vi "Pos ctrl window-Build menu.vi"(8 "error in (no error)":errorcluster) -> (0 "error out":errorcluster, 3 "menu reference out":refnum<k9>)   [LabVIEW 2013]
uses:
  Globals/Pos ctrl window globals.vi
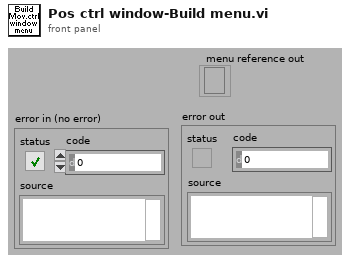
[diagram p1: front panel]
types:
  T1 = typedef "Pos Ctrl window refs cluster.ctl" = cluster{"menu reference":refnum<k9>, "X Coordinate ctrl":refnum<vi>, "Y Coordinate ctrl":refnum<vi>, "Z Coordinate ctrl":refnum<vi>, "Speed setting ctrl":refnum<vi>, "Up":refnum<vi>, "Down":refnum<vi>, "Left":refnum<vi>, "Right":refnum<vi>, "Z move up":refnum<vi>, "Z move down":refnum<vi>, "Down-left":refnum<vi>, "Down-right":refnum<vi>, "Up-left":refnum<vi>, "Up-right":refnum<vi>, "Step = size of image":refnum<vi>, "XY step (um)":refnum<vi>, "Z step (um)":refnum<vi>}
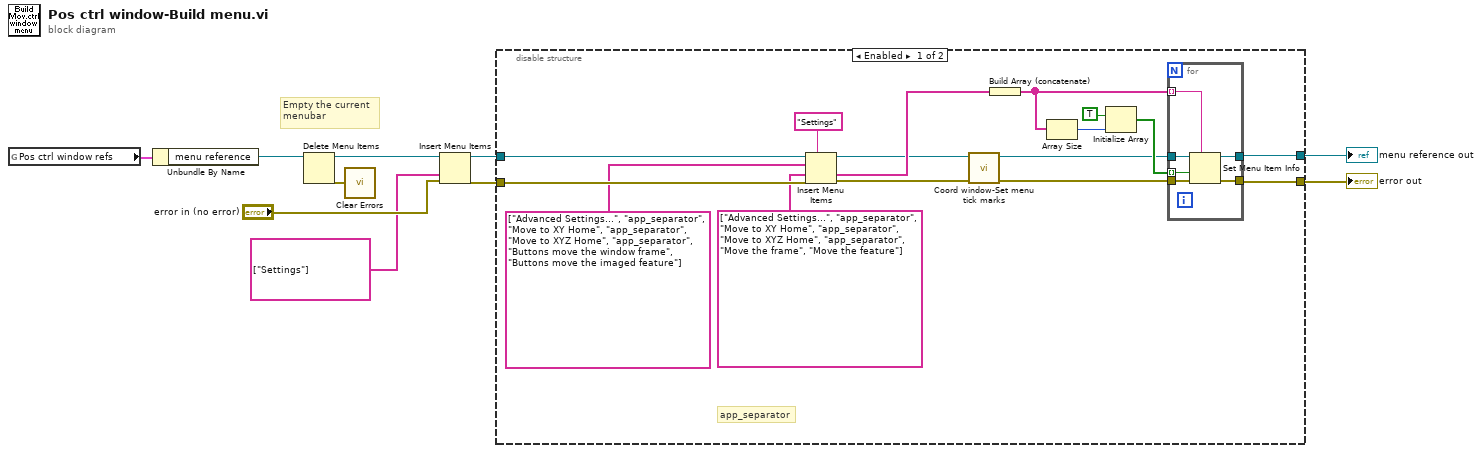
[diagram p0: block diagram]
diagram:
  # "Empty the current\nmenubar"
  n1 = global read "Pos ctrl window globals.vi" "Pos ctrl window refs"() -> (w2:T1)
  n2 = Unbundle By Name(w2) -> ("menu reference"=w1:refnum<k9>)
  n3 = Delete Menu Items(9:w1) -> (0:w5:errorcluster, 3:w8:refnum<k9>)  [unwired: 2 in, 1 out]
  n4 = call <vilib>:"Clear Errors.vi"("error in (no error)"=w5) -> ()  [unwired: 6 in, 1 out]
  n5 = Insert Menu Items(6:"error in (no error)", 7:string[] ["Settings"] ("item tags"), 9:w8) -> (0:w9:errorcluster, 3:w6:refnum<k9>)  [unwired: 4 out]
  n6 = disable-structure shown="Enabled" {
    disable-tunnel: [w26 w33] -> w10
    disable-tunnel: w9 -> [w25 w33]
    disable-tunnel: [w22 w34] -> w7
    disable-tunnel: w6 -> [w20 w34]
    frame Enabled {
      # "app_separator"
      n7 = Insert Menu Items(5:"Settings" ("menu tag"), 6:w25, 7:string[] ["Advanced Settings...", "app_separator", "Move to XY Home", "app_separator", "Move to XYZ Home", "app_separator", "Move the frame", "Move the feature"] ("item tags"), 8:string[] ["Advanced Settings...", "app_separator", "Move to XY Home", "app_separator", "Move to XYZ Home", "app_separator", "Buttons move the window frame", "Buttons move the imaged feature"] ("item tags"), 9:w20) -> (0:w13:errorcluster, 1:w24:string[], 3:w14:refnum<k9>)  [unwired: 1 out]
      n8 = call "Coord window-Set menu tick marks.vi"("error in (no error)"=w13, "Menu in"=w14) -> ("error out"=w12:errorcluster, "Menu out"=w11:refnum<k9>)  [unwired: 8 in]
      n9 = Build Array (concatenate)(w24) -> (w17:string[])
      n10 = Array Size(array=w17) -> (size(s)=w19:i32)
      n11 = Initialize Array(TRUE, w19) -> (w18:bool[])
      n12 = for {
        tunnel: w11 -> [w32]
        tunnel: [w31] -> w22
        tunnel: w17 -> [w30] mode=indexing
        tunnel: w12 -> [w29]
        tunnel: [w28] -> w26
        tunnel: w18 -> [w27] mode=indexing
        n13 = Set Menu Item Info(7:w30, 8:w29, 9:w27, 11:w32) -> (0:w28:errorcluster, 3:w31:refnum<k9>)  [unwired: 1 in, 2 out]
      }
    }
    frame Disabled {
    }
  }
  "error out" <- w10
  "menu reference out" <- w7
